vi "Set Theme.vi"(10 "Boolean":bool, 11 "VI in":refnum<vi>) -> ()   [LabVIEW 2019, in "Panther Dashboard.lvlib"]
uses:
  Panther Dashboard.lvlib
  <vilib>/Utility/miscctls.llb/LVTextColorsTypeDef.ctl
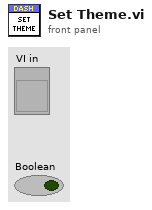
[diagram p1: front panel]
types:
  T1 = typedef "LVTextColorsTypeDef.ctl" = cluster{"Text Color":u32, "Background Color":u32}
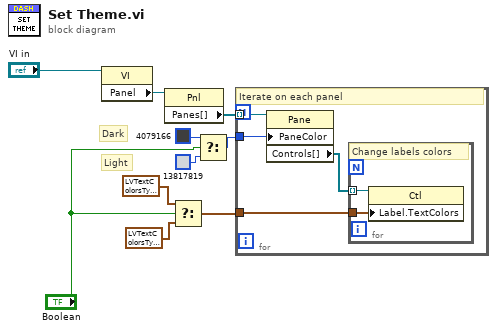
[diagram p0: block diagram]
diagram:
  # "Light"
  # "Dark"
  n1 = property class="VI"(reference="VI in") -> ("Panel"=w4:refnum<vi>)  [unwired: 1 in, 2 out]
  n2 = property class="Pnl"(reference=w4) -> ("Panes[]"=w3:refnum<vi>[])  [unwired: 1 in, 2 out]
  n3 = Select(t=T1 {"Text Color"=16448250, "Background Color"=4079166} ("Label.Text Colors"), s="Boolean", f=T1 {"Text Color"=4079166, "Background Color"=13817819} ("Label.Text Colors")) -> (s? t:f=w1:T1)
  n4 = Select(t=u32 4079166, s="Boolean", f=u32 13817819) -> (s? t:f=w2:u32)
  n5 = for {
    tunnel: w3 -> [w14] mode=indexing
    tunnel: w2 -> [w13]
    tunnel: w1 -> [w11]
    # "Iterate on each panel"
    n6 = property class="Pane"(reference=w14, "PaneColor"=w13) -> ("Controls[]"=w12:refnum<vi>[])  [unwired: 1 in, 2 out]
    n7 = for {
      tunnel: w12 -> [w16] mode=indexing
      tunnel: w11 -> [w15]
      # "Change labels colors"
      n8 = property class="Ctl"(reference=w16, "Label.TextColors"=w15) -> ()  [unwired: 1 in, 2 out]
    }
  }
